vi "AIRobotToSslSimulationProtocolRobot.vi"(8 "error in (no error)":errorcluster, 9 "dribbler_rpm":dbl=1000.0, 10 "Robot":refnum<class "Robot.lvclass">, 11 "Communication in":refnum<class "Communication.lvclass">) -> (0 "error out":errorcluster, 2 "sslSimulationProtocolRobot":T1, 3 "Communication out":refnum<class "Communication.lvclass">)   [LabVIEW 2020, in "Communication.lvclass"]
uses:
  Communication.lvclass
  Robot_class/Robot.lvclass
  Paths/Convert AI Robot to Robot Command Folder/grSim/grSim Robot Command.ctl
  Robot_class/Robot.lvclass/Robot.ctl
  Robot_class/Read id.vi
  Robot_class/Read kick_x.vi
  Robot_class/Read kick_z.vi
  Robot_class/Read v_tang.vi
  Robot_class/Read v_norm.vi
  Robot_class/Read v_ang.vi
  Robot_class/Read dribble.vi
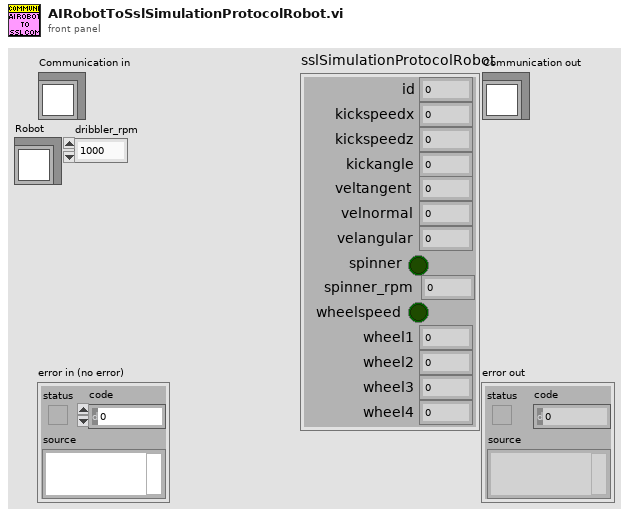
[diagram p1: front panel]
types:
  T1 = typedef "grSim Robot Command.ctl" = cluster{"id":u32, "kickspeedx":sgl, "kickspeedz":sgl, "veltangent":sgl, "velnormal":sgl, "velangular":sgl, "spinner":bool, "wheelspeed":bool, "wheel1":sgl, "wheel2":sgl, "wheel3":sgl, "wheel4":sgl, "kickangle":sgl, "spinner_rpm":sgl}
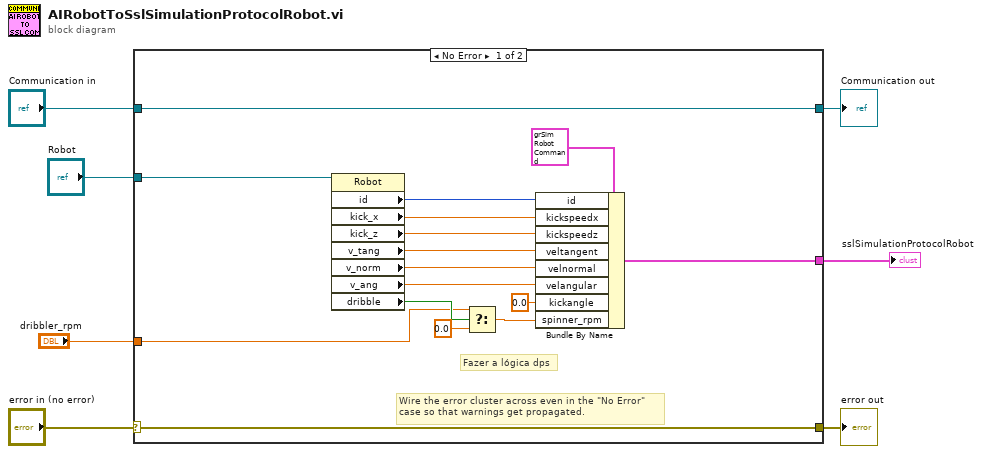
[diagram p0: block diagram]
diagram:
  n1 = case shown="No Error" "error in (no error)" {
    selector: "error in (no error)" -> [w22 w25]
    tunnel: [w22 w25] -> w6
    tunnel: [w23 w24] -> w4
    tunnel: "Communication in" -> [w23 w24]
    tunnel: "Robot" -> [w15 _]
    tunnel: [w13 _] -> w2
    tunnel: "dribbler_rpm" -> [w8 _]
    frame No Error {
      # "Fazer a lógica dps"
      # "Wire the error cluster across even in the \"No Error\"\ncase so that warnings get propagated."
      n2 = property class="Robot"(reference=w15) -> ("id"=w16:i32, "kick_x"=w17:dbl, "kick_z"=w18:dbl, "v_tang"=w19:dbl, "v_norm"=w20:dbl, "v_ang"=w21:dbl, "dribble"=w11:bool)  [unwired: 1 in, 2 out]
      n3 = Select(t=w8, s=w11, f=0.0) -> (s? t:f=w10:dbl)
      n4 = Bundle By Name(cluster=T1 {"id"=0, "kickspeedx"=0.0, "kickspeedz"=0.0, "veltangent"=0.0, "velnormal"=0.0, "velangular"=0.0, "spinner"=FALSE, "wheelspeed"=FALSE, "wheel1"=0.0, "wheel2"=0.0, "wheel3"=0.0, "wheel4"=0.0, "kickangle"=0.0, "spinner_rpm"=0.0} ("grSim Robot Command"), "id"=w16, "kickspeedx"=w17, "kickspeedz"=w18, "veltangent"=w19, "velnormal"=w20, "velangular"=w21, "kickangle"=sgl 0.0, "spinner_rpm"=w10) -> (w13:T1)
    }
    frame Error {
    }
  }
  "error out" <- w6
  "Communication out" <- w4
  "sslSimulationProtocolRobot" <- w2
